vi "XSens VISA to Host (SubVI).vi"(7 "XSense Queue In":refnum<queue>, 8 "error in (no error)":errorcluster, 10 "Serial Settings":T1={"baud rate"=115200, "data bits"=8, "parity"=enum."None", "stop bits"=10, "flow control"=0} {"flow control" items=["None"=0, "XON/XOFF"=1, "RTS/CTS"=2, "DTR/DSR"=4]; "stop bits" items=["1.0"=10, "1.5"=15, "2.0"=20]; "data bits" min=5 max=8 step=1; "baud rate" items=["75"=75, "110"=110, "134"=134, "150"=150, "300"=300, "600"=600, "1200"=1200, "1800"=1800, "2400"=2400, "4800"=4800, "7200"=7200, "9600"=9600, "14400"=14400, "19200"=19200, "28800"=28800, "38400"=38400, "56000"=56000, "57600"=57600, "115200"=115200, "128000"=128000, "230400"=230400]}, 11 "VISA resource name":refnum<visa-resource-name>="ASRL3::INSTR") -> (0 "error out":errorcluster)   [LabVIEW 2019]
doc: "This SubVI reads Xsens data stream from a serial port using VISA. It scans the byte stream one byte at a time to find the MT message header. It rebuilds the data packet header with bytes that were *consumed* as part of this stream screening process. This rebuild is necessary for the checksum process to work. Data are output to a message queue. \n\n2020 NREL"
uses:
  Globals and Definitions/Serial - Settings.ctl
  <vilib>/Instr/_visa.llb/VISA Configure Serial Port (Instr).vi
  Globals and Definitions/RT Globals RD v1.0.vi
panel:
  out "Buffer Dump":string
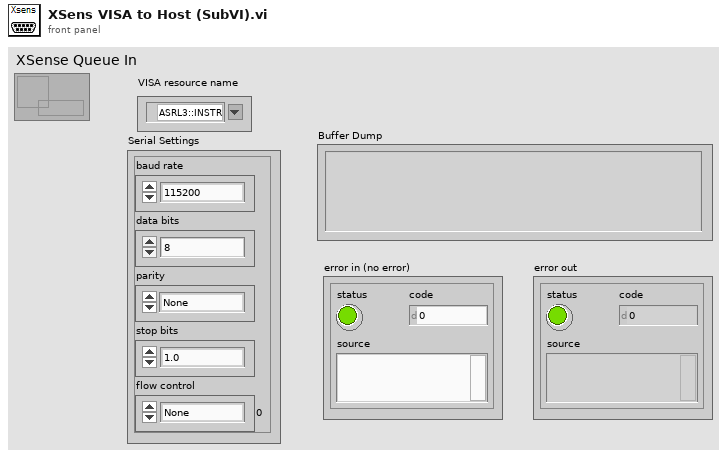
[diagram p1: front panel]
types:
  T1 = typedef "Serial - Settings.ctl" = cluster{"baud rate":u32, "data bits":u16, "parity":enum16{"None", "Odd", "Even", "Mark", "Space"}, "stop bits":u16, "flow control":u16}
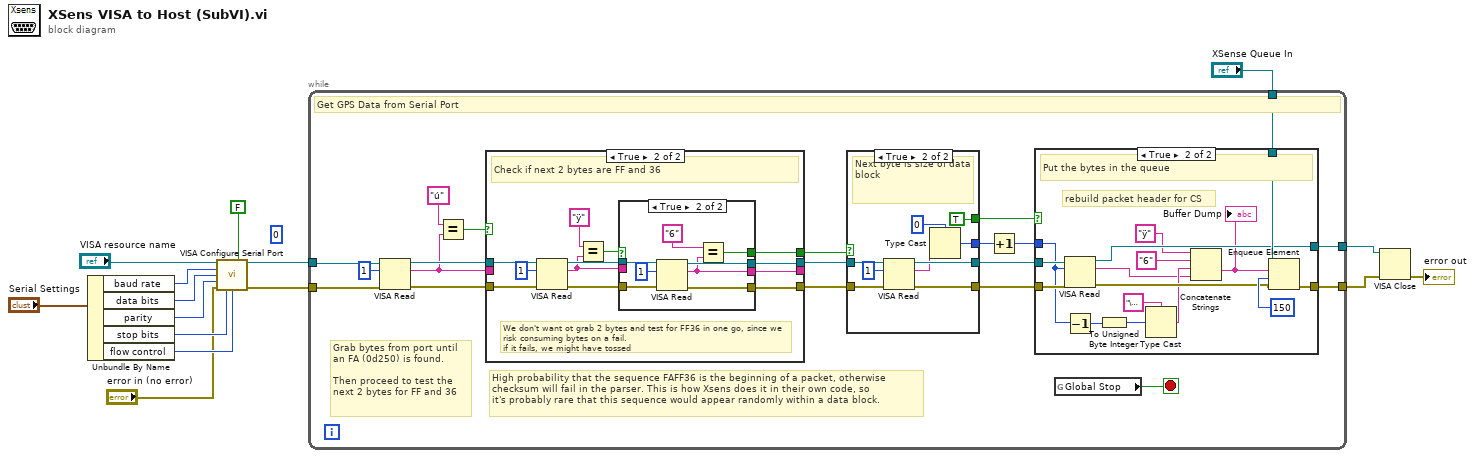
[diagram p0: block diagram]
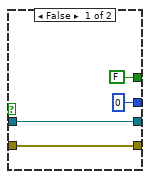
[diagram p3: hidden frame]
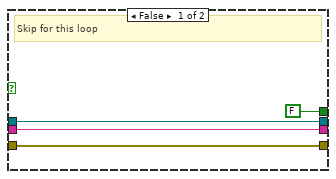
[diagram p4: hidden frame]
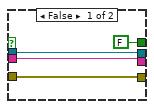
[diagram p5: hidden frame]
diagram:
  (unwired) 0
  n1 = Unbundle By Name("Serial Settings") -> ("baud rate"=w9:u32, "data bits"=w10:u16, "parity"=w11:enum16{"None", "Odd", "Even", "Mark", "Space"}, "stop bits"=w12:u16, "flow control"=w15:u16)
  n2 = call-poly "VISA Configure Serial Port"("VISA resource name"="VISA resource name", "Enable Termination\nChar (T)"=FALSE ("Enable Termination\nChar (T)"), "baud rate (9600)"=w9, "data bits (8)"=w10, "parity (0:none)"=w11, "error in (no error)"="error in (no error)", "stop bits (10: 1 bit)"=w12, "flow control (0:none)"=w15) -> ("VISA resource name out"=w5:refnum<visa-resource-name>, "error out"=w6:errorcluster)  [unwired: 2 in, 4 out]
  n3 = while {
    tunnel: "XSense Queue In" -> [w34]
    tunnel: w6 -> [w32]
    tunnel: w5 -> [w33]
    tunnel: [w31] -> w3
    tunnel: [w16] -> w1
    stop <- w35 stop-if-true
    # "High probability that the sequence FAFF36 is the beginning of a packet, otherwise\nchecksum will fail in the parser. This is how Xsens does it in their own code, so\nit's probably rare that this sequence would appear randomly within a data block."
    # "Grab bytes from port until\nan FA (0d250) is found.\n\nThen proceed to test the \nnext 2 bytes for FF and 36"
    # "Get GPS Data from Serial Port"
    n4 = VISA Read(VISA resource name=w33, byte count=u32 1, error in (no error)=w32) -> (VISA resource name out=w28:refnum<visa-resource-name>, read buffer=w26:string, error out=w27:errorcluster)  [unwired: 1 out]
    n5 = Equal?(x="ú", y=w26) -> (x = y?=w29:bool)
    n6 = case shown="True" w29 {
      tunnel: w28 -> [w69 w82]
      tunnel: w27 -> [w70 w81]
      tunnel: [w69 w75] -> w24
      tunnel: [w70 w74] -> w23
      tunnel: [w68 w73] -> _
      tunnel: w26 -> [w68 _]
      tunnel: [FALSE w71] -> w25
      frame False {
        # "Skip for this loop"
      }
      frame True {
        # "We don't want ot grab 2 bytes and test for FF36 in one go, since we risk consuming bytes on a fail.\nif it fails, we might have tossed"
        # "Check if next 2 bytes are FF and 36"
        n7 = VISA Read(VISA resource name=w82, byte count=u32 1, error in (no error)=w81) -> (VISA resource name out=w77:refnum<visa-resource-name>, read buffer=w72:string, error out=w76:errorcluster)  [unwired: 1 out]
        n8 = Equal?(x="ÿ", y=w72) -> (x = y?=w78:bool)
        n9 = case shown="True" w78 {
          tunnel: w77 -> [w85 w92]
          tunnel: w76 -> [w84 w91]
          tunnel: [w85 w90] -> w75
          tunnel: [w84 w89] -> w74
          tunnel: [w86 w88] -> w73
          tunnel: w72 -> [w86 _]
          tunnel: [FALSE w87] -> w71
          frame False {
          }
          frame True {
            n10 = VISA Read(VISA resource name=w92, byte count=u32 1, error in (no error)=w91) -> (VISA resource name out=w90:refnum<visa-resource-name>, read buffer=w88:string, error out=w89:errorcluster)  [unwired: 1 out]
            n11 = Equal?(x="6", y=w88) -> (x = y?=w87:bool)
          }
        }
      }
    }
    n12 = case shown="True" w25 {
      tunnel: w24 -> [w56 w65]
      tunnel: w23 -> [w57 w64]
      tunnel: [w56 w63] -> w17
      tunnel: [w57 w62] -> w18
      tunnel: [u8 0 ("default (0 U32)") w59] -> w20
      tunnel: [FALSE TRUE] -> w21
      frame False {
      }
      frame True {
        # "Next byte is size of data block"
        n13 = VISA Read(VISA resource name=w65, byte count=u32 1, error in (no error)=w64) -> (VISA resource name out=w63:refnum<visa-resource-name>, read buffer=w61:string, error out=w62:errorcluster)  [unwired: 1 out]
        n14 = Type Cast(type=u8 0 ("default (0 U32)"), x=w61) -> (*(type *) &x=w59:u8)
      }
    }
    n15 = Increment(x=w20) -> (x+1=w19:u8)
    n16 = case shown="True" w21 {
      tunnel: w34 -> [_ w53]
      tunnel: [w36 w51] -> w31
      tunnel: w19 -> [_ w43]
      tunnel: w18 -> [w36 w50]
      tunnel: w17 -> [w37 w49]
      tunnel: [w37 w47] -> w16
      frame False {
      }
      frame True {
        # "rebuild packet header for CS"
        # "Put the bytes in the queue"
        n17 = VISA Read(VISA resource name=w49, byte count=w43, error in (no error)=w50) -> (VISA resource name out=w47:refnum<visa-resource-name>, read buffer=w39:string, error out=w48:errorcluster)  [unwired: 1 out]
        n18 = Decrement(x=w43) -> (x-1=w46:u8)
        n19 = To Unsigned Byte Integer(number=w46) -> (unsigned 8bit integer=w45:u8)
        n20 = Type Cast(type="\u0000" ("name (unnamed)"), x=w45) -> (*(type *) &x=w40:string)
        n21 = Concatenate Strings("ÿ" ("name (unnamed)"), "6" ("name (unnamed)"), w40, w39) -> (w38:string)
        "Buffer Dump" <- w38
        n22 = Enqueue Element(queue=w53, element=w38, timeout in ms (-1)=150, error in (no error)=w48) -> (error out=w51:errorcluster)  [unwired: 2 out]
      }
    }
    n23 = global read "RT Globals RD v1.0.vi" "Global Stop"() -> (w35:bool)
  }
  n24 = VISA Close(VISA resource name=w1, error in (no error)=w3) -> (error out=→"error out":errorcluster)
